vi "Exercise 3.3 User-controlled Filter.vi"() -> ()   [LabVIEW 2024]
uses:
  <vilib>/express/express analysis/Spectral/Block/exnSpectralBlock spectral measurements RMS poly.vi
  <vilib>/express/express analysis/Spectral/Block/exnSpectralBlock spectral measurements RMS DDT.vi
  <vilib>/express/express analysis/Spectral/XNode/ExpressSpectralMeasurementsBlockNode.xnode
panel:
  in  "Upper":dbl(slide) scale=0.0..700.0
  out "Det. Peak":dbl
  out "FFT(RMS)":dynamicdata(graph)
  out "Over  Limit?":bool
  in  "stop":bool
  in  "Lower Limit":dbl(knob) scale=0.0..500.0
  in  "Upper Limit":dbl(knob) scale=0.0..2000.0
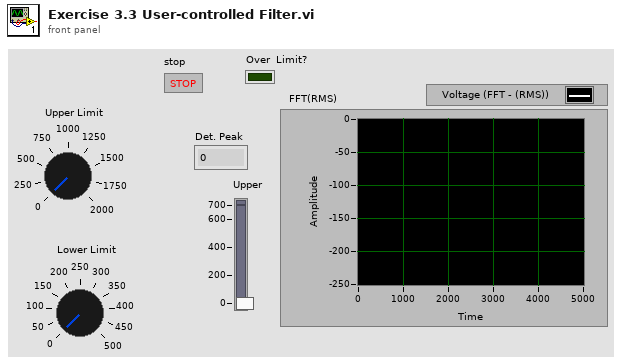
[diagram p1: front panel]
types:
  T1 = cluster{"averaging mode":u16, "weighting mode":u16, "number of averages":u32}
  T2 = cluster{"dB On (F)":bool, "unwrap phase (F)":bool, "convert to degree (F)":bool}
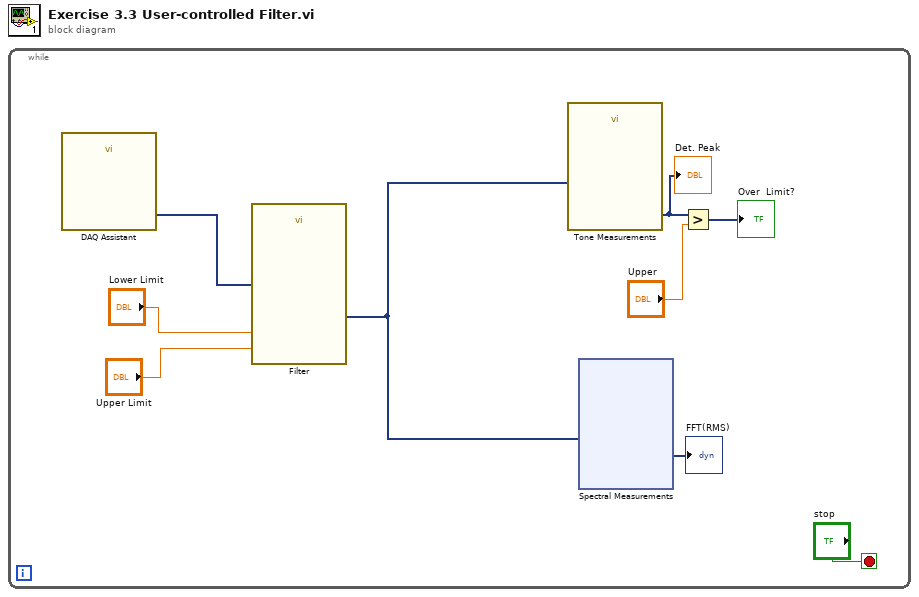
[diagram p0: block diagram]
diagram:
  n1 = while {
    stop <- "stop" stop-if-true
    n2 = call "DAQ Assistant"() -> ("data"=w9:dynamicdata)  [unwired: 16 in, 3 out]
    n3 = call "Filter"("Lower Cut-Off"="Lower Limit", "Upper Cut-Off"="Upper Limit", "Signal"=w9) -> ("Filtered Signal"=w5:dynamicdata)  [unwired: 7 in, 1 out]
    n4 = call "Tone Measurements"("Signals"=w5) -> ("Frequency"=w2:dynamicdata)  [unwired: 8 in, 2 out]
    "Det. Peak" <- w2
    n5 = xnode "Spectral Measurements"("Signals"=w5) -> ("FFT - (RMS)"=→"FFT(RMS)":dynamicdata)  [unwired: 1 in, 2 out]
    n6 = Greater?(x=w2, y="Upper") -> (0:→"Over  Limit?":dynamicdata)
  }
